vi "detect stack cube.vi"() -> (0 "Type":enum16{"Z", "I", "O", "S", "L", "J", "T", "N"}(ring))   [LabVIEW 2018]
uses:
  Vision info.vi
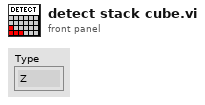
[diagram p1: front panel]
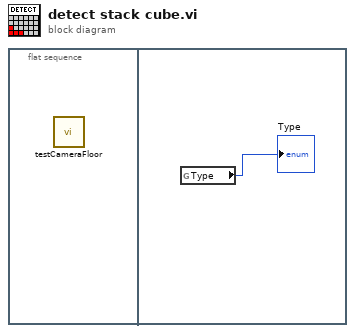
[diagram p0: block diagram]
diagram:
  n1 = flat-sequence {
    frame #0 {
      n2 = call "testCameraFloor.vi"() -> ()  [unwired: 12 in]
    }
    frame #1 {
      n3 = global read "Vision info.vi" "Type"() -> (→"Type":enum16{"Z", "I", "O", "S", "L", "J", "T", "N"})
    }
  }
